vi "InitCamera.vi"(11 "Camera ID":u32) -> (0 "error out":errorcluster, 3 "Camera Handle Out":u32)   [LabVIEW 2011]
doc: "InitCamera opens the driver and connects to the hardware.\n\nCamera ID indicates the ID of the camera, which is to be opened.\nAt the value \"0\" the first not opened camera is used."
uses:
  uEye_api.dll
panel:
  # "Input"
  # "Output"
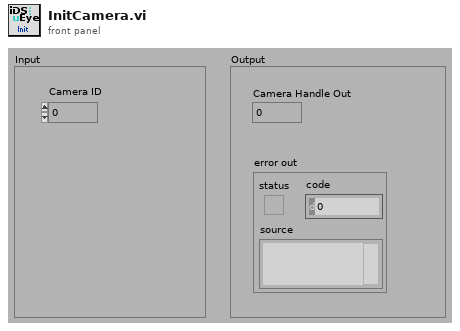
[diagram p1: front panel]
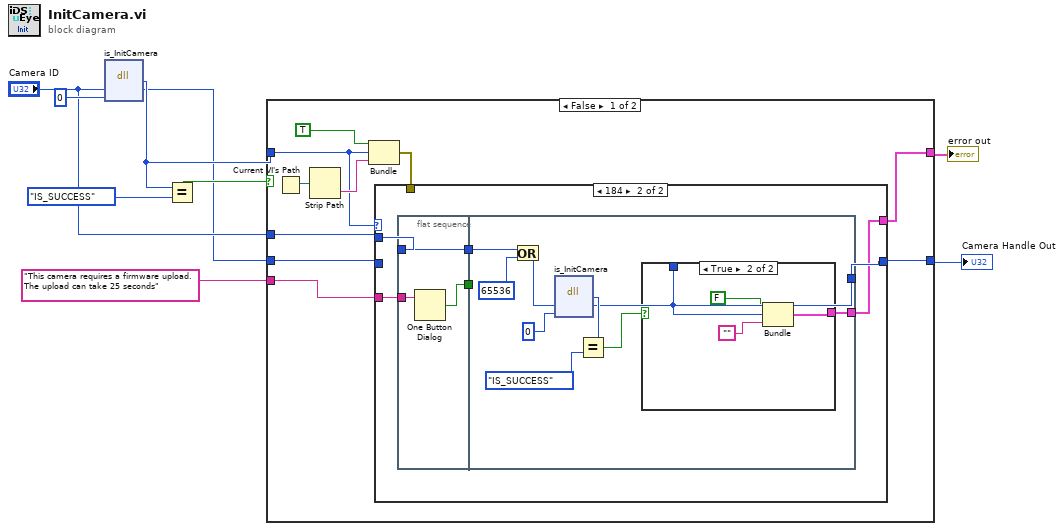
[diagram p0: block diagram]
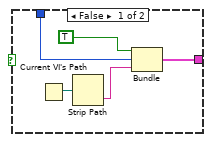
[diagram p3: hidden frame]
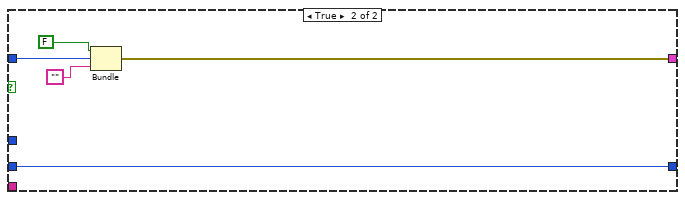
[diagram p4: hidden frame]
diagram:
  n1 = dll-call lib="uEye_api.dll" fn="is_InitCamera"("phf"="Camera ID", "hWnd"=0) -> (w6:i32, "phf"=w3:u32)  [unwired: 4 in, 2 out]
  n2 = Equal?(x=w6, y=enum16{"IS_SUCCESS"}."IS_SUCCESS") -> (x = y?=w7:bool)
  n3 = case shown="False" w7 {
    tunnel: [w14 w50] -> w5
    tunnel: w6 -> [w16 w53]
    tunnel: "Camera ID" -> [w13 _]
    tunnel: w3 -> [w12 w49]
    tunnel: [w11 w49] -> w2
    tunnel: "This camera requires a firmware upload. The upload can take 25 seconds" ("Nachricht") -> [w10 _]
    frame False {
      n4 = Current VI's Path() -> (path=w18:path)
      n5 = Strip Path(path=w18) -> (name=w17:string)  [unwired: 1 out]
      n6 = Bundle(TRUE, w16, "name"=w17) -> (w15:cluster{bool, i32, "name":string})  [unwired: 1 in]
      n7 = case shown="184" w16 {
        tunnel: w15 -> [w21 _]
        tunnel: [w21 w23] -> w14
        tunnel: w13 -> [_ w27]
        tunnel: w12 -> [w20 _]
        tunnel: [w20 w24] -> w11
        tunnel: w10 -> [_ w22]
        frame Default {
        }
        frame 184 {
          n8 = flat-sequence {
            tunnel: w27 -> [w30]
            tunnel: [w30] -> w26
            tunnel: [w29] -> w25
            tunnel: w22 -> [w28]
            tunnel: w26 -> [w33]
            tunnel: w25 -> [_]
            tunnel: [w36] -> w24
            tunnel: [w35] -> w23
            frame #0 {
              n9 = One Button Dialog(message=w28) -> (true=w29:bool)  [unwired: 1 in]
            }
            frame #1 {
              n10 = Or(x=w33, y=u32 65536) -> (x .or. y?=w31:u32)
              n11 = dll-call lib="uEye_api.dll" fn="is_InitCamera"("phf"=w31, "hWnd"=0) -> (w38:i32, "phf"=w36:u32)  [unwired: 4 in, 2 out]
              n12 = Equal?(x=w38, y=enum16{"IS_SUCCESS"}."IS_SUCCESS") -> (x = y?=w37:bool)
              n13 = case shown="True" w37 {
                tunnel: w36 -> [w42 w45]
                tunnel: [w40 w46] -> w35
                frame False {
                  n14 = Current VI's Path() -> (path=w43:path)
                  n15 = Strip Path(path=w43) -> (name=w41:string)  [unwired: 1 out]
                  n16 = Bundle(TRUE, "phf"=w42, "name"=w41) -> (w40:cluster{bool, "phf":u32, "name":string})  [unwired: 1 in]
                }
                frame True {
                  n17 = Bundle(FALSE, "phf"=w45, "") -> (w46:cluster{bool, "phf":u32, string})  [unwired: 1 in]
                }
              }
            }
          }
        }
      }
    }
    frame True {
      n18 = Bundle(FALSE, w53, "") -> (w50:errorcluster)  [unwired: 1 in]
    }
  }
  "Camera Handle Out" <- w2
  "error out" <- w5
